vi "Open Audio File Write (WAV).vi"(8 "error in (no error)":errorcluster, 9 "Codec Specific Info":T1={"Container Format"=enum."RIFF", "Data Format"=1} {"Data Format" items=["PCM"=1, "ADPCM"=2, "IEEE Float"=3]}, 10 "Audio File Info":T4={"Sample Rate (Hz)"=44100, "Channels"=2, "Bit Depth"=16}, 11 "Path":path) -> (0 "error out":errorcluster, 3 "Audio File Refnum":T5)   [LabVIEW 2020, in "G-Audio.lvlib"]
doc: "Create or replace an audio file and initialize the WAV encoder for writing."
uses:
  G-Audio.lvlib
  Controls/Audio File Refnum.ctl
  Controls/Audio File Info.ctl
  Controls/WAV Codec Specific Info.ctl
  Controls/WAV Container Format.ctl
  Controls/WAV Data Format.ctl
  Private/Result To Error.vi
  <vilib>/Utility/error.llb/Error Cluster From Error Code.vi
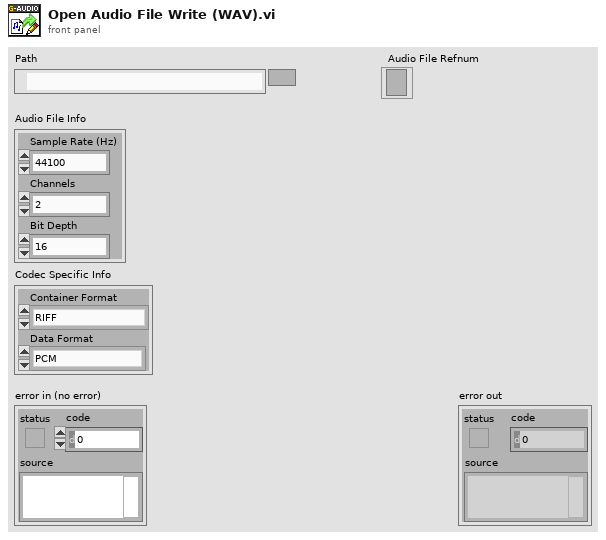
[diagram p1: front panel]
types:
  T1 = typedef "G-Audio.lvlib/WAV Codec Specific Info.ctl" = cluster{"Container Format":T2, "Data Format":T3}
  T2 = typedef "G-Audio.lvlib/WAV Container Format.ctl" = enum32{"RIFF", "Wave64"}
  T3 = typedef "G-Audio.lvlib/WAV Data Format.ctl" = u32
  T4 = typedef "G-Audio.lvlib/Audio File Info.ctl" = cluster{"Sample Rate (Hz)":u32, "Channels":u32, "Bit Depth":u32}
  T5 = typedef "G-Audio.lvlib/Audio File Refnum.ctl" = refnum<file>
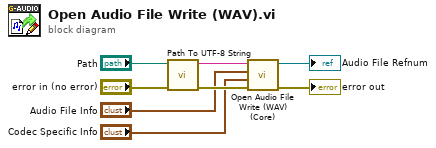
[diagram p0: block diagram]
diagram:
  n1 = call "Path To UTF-8 String.vi"("error in"="error in (no error)", "Path"="Path") -> ("error out"=w5:errorcluster, "UTF-8 String"=w8:string)  [unwired: 8 in]
  n2 = call "Open Audio File Write (WAV) (Core).vi"("error in (no error)"=w5, "Codec Specific Info"="Codec Specific Info", "Audio File Info"="Audio File Info", "Path"=w8) -> ("error out"=→"error out":errorcluster, "Audio File Refnum"=→"Audio File Refnum":T5)  [unwired: 6 in]
